vi "XtoY.vi"(1 "x":dbl[](array[numeric])=[1.0, -2.0, 3.0, -4.0, 5.0] format="%.2e", 2 "y":i32) -> (0 "x^y":dbl[](array[numeric])=[1.0, 1.0, 1.0, 1.0, 1.0] format="%.2e")   [LabVIEW 2014]
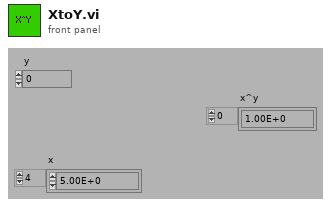
[diagram p1: front panel]
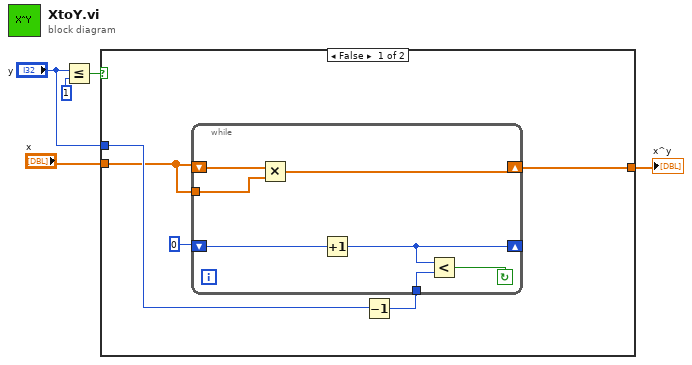
[diagram p0: block diagram]
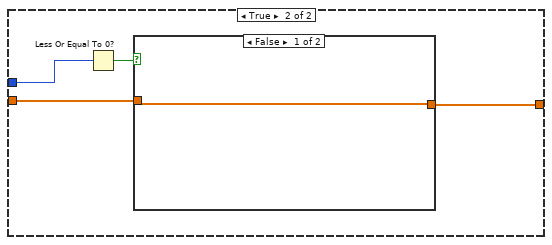
[diagram p2: hidden frame]
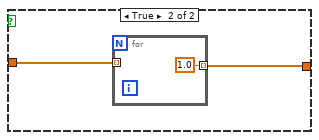
[diagram p3: hidden frame]
diagram:
  n1 = Less Or Equal?(x="y", y=1) -> (x <= y?=w5:bool)
  n2 = case shown="False" w5 {
    tunnel: "y" -> [w7 w20]
    tunnel: [w8 w19] -> w1
    tunnel: "x" -> [w6 w18]
    frame False {
      n3 = Decrement(x=w7) -> (x-1=w10:i32)
      n4 = while {
        tunnel: w6 -> [w11]
        shift-left: w6 -> [w15]
        shift-right: [w14] -> w8
        tunnel: w10 -> [w16]
        shift-left: 0 -> [w13]
        shift-right: [w12] -> _
        stop <- w17 continue-if-true
        n5 = Multiply(x=w15, y=w11) -> (x*y=w14:dbl[])
        n6 = Increment(x=w13) -> (x+1=w12:i32)
        n7 = Less?(x=w12, y=w16) -> (x < y?=w17:bool)
      }
    }
    frame True {
      n8 = Less Or Equal To 0?(x=w20) -> (x <= 0?=w21:bool)
      n9 = case shown="False" w21 {
        tunnel: [w22 w23] -> w19
        tunnel: w18 -> [w22 w24]
        frame False {
        }
        frame True {
          n10 = for {
            tunnel: w24 -> [_] mode=indexing
            tunnel: [1.0] -> w23 mode=indexing
          }
        }
      }
    }
  }
  "x^y" <- w1
